vi "Analyze.vi"(8 "error in (no error)":errorcluster, 9 "Work Image":T1, 10 "Destination":refnum<class "Message Enqueuer.lvclass">, 11 "Analyze Data":T2) -> (0 "error out":errorcluster)   [LabVIEW 2020, in "Analyze Actor.lvlib" / "Analyze Actor.lvclass"]
uses:
  Analyze Actor.lvclass
  Display Actors/HIJ Vision Display/HIJ Vision Display/Analyze.ctl
  <vilib>/vision/Image Controls.llb/IMAQ Image.ctl
  <vilib>/ActorFramework/Message Enqueuer/Message Enqueuer.lvclass
  Abstract Messages/Publish Analyze Results Msg/Publish Analyze Results Msg.lvclass/Publish Analyze Results Msg.ctl
  <vilib>/ActorFramework/Message Enqueuer/Message Enqueuer.lvclass/Message Enqueuer.ctl
  <vilib>/ActorFramework/Message Enqueuer/Enqueue.vi
  <vilib>/ActorFramework/Message Priority Queue/Priority Enqueue.vi
  Analyze Actor.lvclass/Analyze Actor.ctl
  Analyze Classes/Analyze BaseClass/Analyze BaseClass/Analyze BaseClass.lvclass
  IAnalysis Messages/Analysis Results Msg/Analysis Results Msg.lvclass
  Results and Overlays/Results Base/Analyze Results Base.lvclass
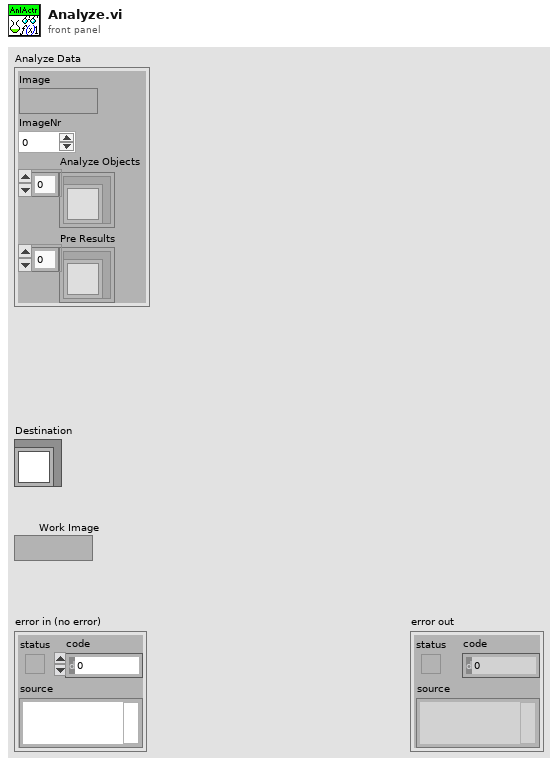
[diagram p1: front panel]
types:
  T1 = typedef "IMAQ Image.ctl" = refnum<image>
  T2 = typedef "Analyze Actor.lvlib/Analyze Actor.lvclass/Analyze.ctl" = cluster{"Image":T1, "ImageNr":i32, "Analyze Objects":refnum<class "Analyze BaseClass.lvclass">[], "Pre Results":refnum<class "Analyze Results Base.lvclass">[]}
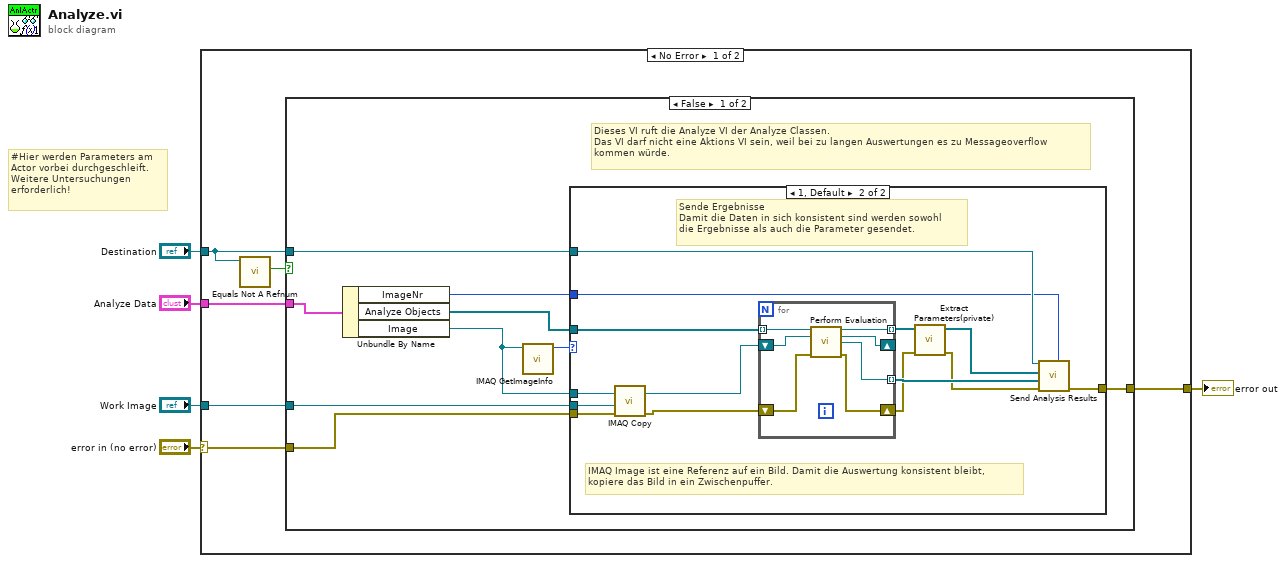
[diagram p0: block diagram]
diagram:
  # "#Hier werden Parameters am\nActor vorbei durchgeschleift.\nWeitere Untersuchungen \nerforderlich!"
  n1 = case shown="No Error" "error in (no error)" {
    selector: "error in (no error)" -> [w11 w44]
    tunnel: [w9 w44] -> w4
    tunnel: "Analyze Data" -> [w10 _]
    tunnel: "Destination" -> [w8 _]
    tunnel: "Work Image" -> [w6 _]
    frame No Error {
      n2 = call <vilib>:"Equals Not A Refnum.vi"("Message Enqueuer"=w8) -> ("Not a refnum?"=w7:bool)  [unwired: 10 in]
      n3 = case shown="False" w7 {
        tunnel: w11 -> [w15 w43]
        tunnel: w10 -> [w20 _]
        tunnel: [w18 w43] -> w9
        tunnel: w8 -> [w17 _]
        tunnel: w6 -> [w16 _]
        frame False {
          # "Dieses VI ruft die Analyze VI der Analyze Classen.\nDas VI darf nicht eine Aktions VI sein, weil bei zu langen Auswertungen es zu Messageoverflow\nkommen würde."
          n4 = Unbundle By Name(w20) -> ("ImageNr"=w12:i32, "Analyze Objects"=w19:refnum<class "Analyze BaseClass.lvclass">[], "Image"=w14:T1)
          n5 = call "IMAQ GetImageInfo"("Image"=w14) -> ("X Resolution"=w13:i32)  [unwired: 3 in, 7 out]
          n6 = case shown="1, Default" w13 {
            tunnel: w19 -> [_ w35]
            tunnel: [w21 w34] -> w18
            tunnel: w17 -> [_ w33]
            tunnel: w16 -> [_ w32]
            tunnel: w15 -> [w21 w31]
            tunnel: w12 -> [_ w22]
            tunnel: w14 -> [_ w23]
            frame 0 {
            }
            frame 1, Default {
              # "Sende Ergebnisse\nDamit die Daten in sich konsistent sind werden sowohl\ndie Ergebnisse als auch die Parameter gesendet."
              # "IMAQ Image ist eine Referenz auf ein Bild. Damit die Auswertung konsistent bleibt,\nkopiere das Bild in ein Zwischenpuffer."
              n7 = call "IMAQ Copy"("error in (no error)"=w31, "Image Dst"=w32, "Image Src"=w23) -> ("error out"=w30:errorcluster, "Image Dst Out"=w29:T1)  [unwired: 3 in]
              n8 = for {
                tunnel: w35 -> [w41] mode=indexing
                shift-right: [w40] -> _
                shift-left: w29 -> [w42]
                shift-right: [w37] -> w26
                shift-left: w30 -> [w39]
                tunnel: [w38] -> w28 mode=indexing
                tunnel: [w36] -> w27 mode=indexing
                n9 = call "Perform Evaluation.vi"("Analyze BaseClass in"=w41, "Image in"=w42, "error in (no error)"=w39) -> ("Analyze BaseClass out"=w36:refnum<class "Analyze BaseClass.lvclass">, "Image out"=w40:T1, "Result"=w38:refnum<class "Analyze Results Base.lvclass">, "error out"=w37:errorcluster)  [unwired: 9 in]
              }
              n10 = call "Extract Parameters(private).vi"("error in"=w26, "Analyze objs"=w27) -> ("error out"=w25:errorcluster, "Parameters"=w24:refnum<class "Analyze Parameter Base.lvclass">[])  [unwired: 8 in]
              n11 = call "Send Analysis Results.vi"("Image Nr."=w22, "error in (no error)"=w25, "Results In"=w28, "Parameters"=w24, "Message Enqueuer"=w33) -> ("error out"=w34:errorcluster)  [unwired: 5 in, 1 out]
            }
          }
        }
        frame True {
        }
      }
    }
    frame Error {
    }
  }
  "error out" <- w4
